vi "Check Health.vi"(8 "error in (no error)":errorcluster, 10 "Drop Out Value":i32, 11 "Sensor in":refnum<class "Sensor.lvclass">) -> (0 "error out":errorcluster, 2 "Sensor Health":bool, 3 "Sensor out":refnum<class "Sensor.lvclass">)   [LabVIEW 2014, in "Sensors.lvlib" / "Sensor.lvclass"]
uses:
  Sensor.lvclass
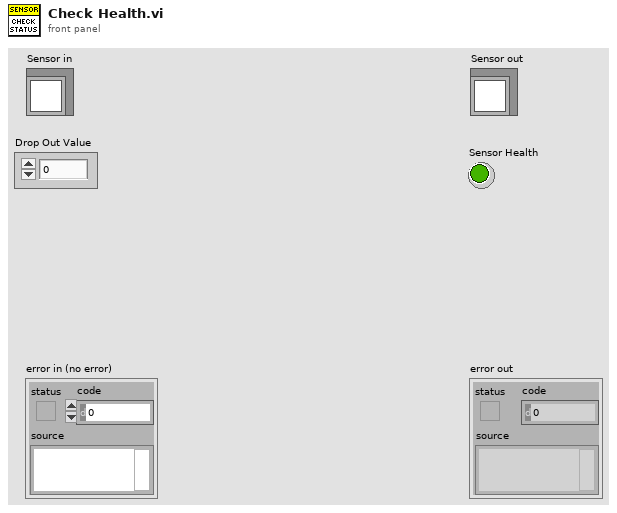
[diagram p1: front panel]
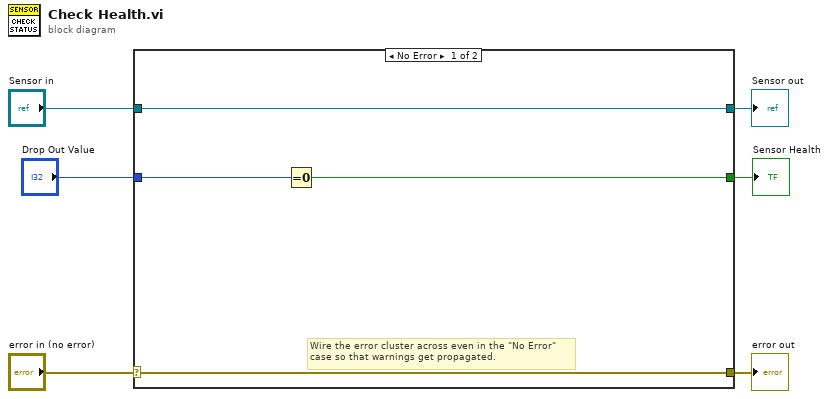
[diagram p0: block diagram]
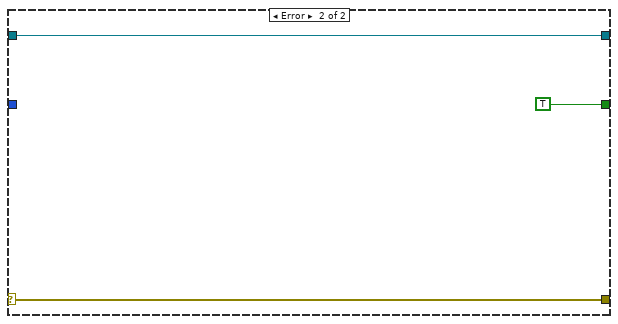
[diagram p2: hidden frame]
diagram:
  n1 = case shown="No Error" "error in (no error)" {
    selector: "error in (no error)" -> [w10 w13]
    tunnel: [w10 w13] -> w5
    tunnel: [w8 w12] -> w3
    tunnel: "Sensor in" -> [w8 w12]
    tunnel: [w9 TRUE] -> w2
    tunnel: "Drop Out Value" -> [w7 _]
    frame No Error {
      # "Wire the error cluster across even in the \"No Error\"\ncase so that warnings get propagated."
      n2 = Equal To 0?(x=w7) -> (x = 0?=w9:bool)
    }
    frame Error {
    }
  }
  "error out" <- w5
  "Sensor out" <- w3
  "Sensor Health" <- w2
